vi "Actuators Move Relative.vi"(0 "Notifier Name":string, 2 "Wait to Finish":bool, 5 "Channel":i32[](array[numeric]), 7 "Step":dbl[](array[numeric]), 11 "Error In":errorcluster) -> (4 "Notifier Name Out":string, 15 "Error Out":errorcluster)   [LabVIEW 2020]
uses:
  Actuators Controls/Actuators Note Type.ctl
  Actuators Controls/Actuators Actions.ctl
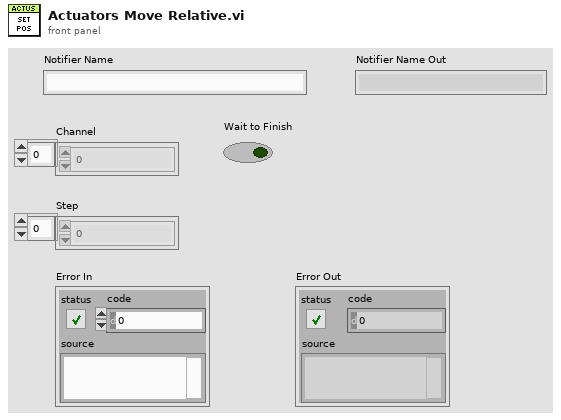
[diagram p1: front panel]
types:
  T1 = typedef "Actuators Note Type.ctl" = cluster{"Actions":T2, "Cmd Received ":bool, "Setpoint":dbl[], "Position":dbl[], "Channel":i32[], "Jog Step":dbl[], "Velocity":dbl[], "Acceleration":dbl[]}
  T2 = typedef "Actuators Actions.ctl" = enum16{"Nothing", "Get Position", "Get Acceleration", "Get Velocity", "Get Jog Step", "Set Acceleration", "Set Velocity", "Set Jog Step", "Move Absolute", "Move Relative", "Jog Forward", "Jog Reverse", "Halt", "Quit"}
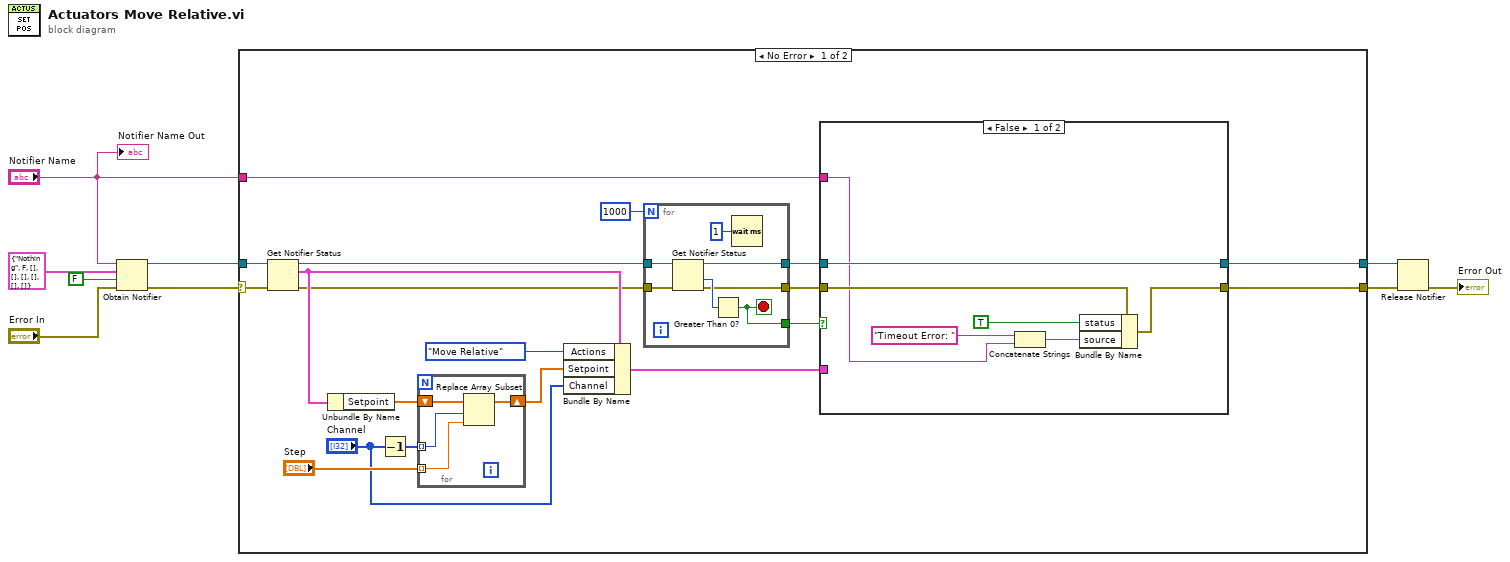
[diagram p0: block diagram]
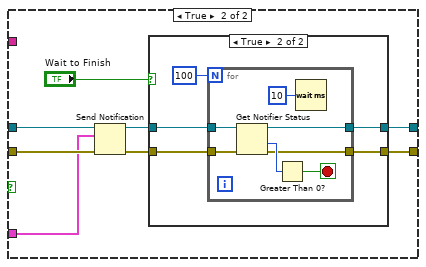
[diagram p2: hidden frame]
diagram:
  n1 = Obtain Notifier(name (unnamed)="Notifier Name", notification data type=T1 {"Actions"=enum."Nothing", "Cmd Received "=FALSE, "Setpoint"=[], "Position"=[], "Channel"=[], "Jog Step"=[], "Velocity"=[], "Acceleration"=[]} ("Actuators Note"), create if not found? (T)=FALSE, error in (no error)="Error In") -> (notifier out=w5:refnum<notifier>, error out=w8:errorcluster)  [unwired: 1 out]
  n2 = case shown="No Error" w8 {
    selector: w8 -> [w19 w69]
    tunnel: w5 -> [w20 w70]
    tunnel: "Notifier Name" -> [w10 _]
    tunnel: [w28 w70] -> w4
    tunnel: [w27 w69] -> w3
    frame No Error {
      n3 = Get Notifier Status(notifier=w20, error in (no error)=w19) -> (notifier out=w16:refnum<notifier>, current notification=w18:T1, error out=w15:errorcluster)  [unwired: 2 out]
      n4 = Unbundle By Name(w18) -> ("Setpoint"=w22:dbl[])
      n5 = Decrement(x="Channel") -> (x-1=w24:i32[])
      n6 = for {
        tunnel: w24 -> [w68] mode=indexing
        tunnel: "Step" -> [w67] mode=indexing
        shift-right: [w65] -> w23
        shift-left: w22 -> [w66]
        n7 = Replace Array Subset(array=w66, new element=w67, index=w68) -> (w65:dbl[])
      }
      n8 = Bundle By Name(cluster=w18, "Actions"=Actuators_Actions."Move Relative", "Setpoint"=w23, "Channel"="Channel") -> (w11:T1)
      n9 = for {
        N: 1000 -> [_]
        tunnel: w16 -> [w64]
        tunnel: [w63] -> w14
        tunnel: w15 -> [w60]
        tunnel: [w59] -> w12
        tunnel: [w58] -> w13
        stop <- w59 stop-if-true
        n10 = Get Notifier Status(notifier=w64, error in (no error)=w60) -> (notifier out=w63:refnum<notifier>, # waiting=w62:i32, error out=w58:errorcluster)  [unwired: 2 out]
        n11 = Greater Than 0?(x=w62) -> (x > 0?=w59:bool)
        n12 = Wait (ms)(milliseconds to wait=u32 1) -> ()  [unwired: 1 out]
      }
      n13 = case shown="False" w12 {
        tunnel: [w30 w43] -> w28
        tunnel: [w31 w42] -> w27
        tunnel: w14 -> [w30 w38]
        tunnel: w13 -> [w32 w37]
        tunnel: w11 -> [_ w36]
        tunnel: w10 -> [w29 _]
        frame False {
          n14 = Concatenate Strings("Timeout Error: " ("source"), w29) -> (w35:string)
          n15 = Bundle By Name(cluster=w32, "status"=TRUE, "source"=w35) -> (w31:errorcluster)
        }
        frame True {
          n16 = Send Notification(notification=w36, notifier=w38, error in (no error)=w37) -> (notifier out=w41:refnum<notifier>, error out=w40:errorcluster)
          n17 = case shown="True" "Wait to Finish" {
            tunnel: w41 -> [w45 w49]
            tunnel: w40 -> [w44 w48]
            tunnel: [w44 w47] -> w42
            tunnel: [w45 w46] -> w43
            frame False {
            }
            frame True {
              n18 = for {
                N: 100 -> [_]
                tunnel: w49 -> [w57]
                tunnel: [w56] -> w46
                tunnel: w48 -> [w53]
                tunnel: [w51] -> w47
                stop <- w52 stop-if-true
                n19 = Get Notifier Status(notifier=w57, error in (no error)=w53) -> (notifier out=w56:refnum<notifier>, # waiting=w55:i32, error out=w51:errorcluster)  [unwired: 2 out]
                n20 = Greater Than 0?(x=w55) -> (x > 0?=w52:bool)
                n21 = Wait (ms)(milliseconds to wait=u32 10) -> ()  [unwired: 1 out]
              }
            }
          }
        }
      }
    }
    frame Error {
    }
  }
  n22 = Release Notifier(notifier=w4, error in (no error)=w3) -> (error out=→"Error Out":errorcluster)  [unwired: 1 in, 2 out]
  "Notifier Name Out" <- "Notifier Name"
